vi "ButtonRaiseStack.vi"(11 "Buttons":bool[](array[boolean])) -> ()   [LabVIEW 2014]
uses:
  Gantry/GantryGlobals.vi
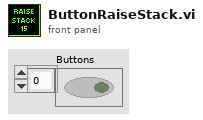
[diagram p1: front panel]
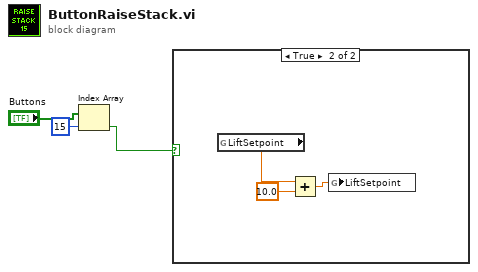
[diagram p0: block diagram]
diagram:
  n1 = Index Array(array="Buttons", index=15) -> (element=w1:bool)
  n2 = case shown="True" w1 {
    frame False {
    }
    frame True {
      n3 = global read "GantryGlobals.vi" "LiftSetpoint"() -> (w5:dbl)
      n4 = Add(x=w5, y=10.0) -> (x+y=w6:dbl)
      n5 = global write "GantryGlobals.vi" "LiftSetpoint"(w6) -> ()
    }
  }
